vi "Release.vi"(8 "error in (no error)":errorcluster, 11 "SequenceCountService in":refnum<class "SequenceCountService.lvclass">) -> (0 "error out":errorcluster)   [LabVIEW 2020, in "Vecto.lvlib" / "SequenceCountService.lvclass"]
uses:
  SequenceCountService.lvclass
  SequenceCountService.lvclass/SequenceCountService.ctl
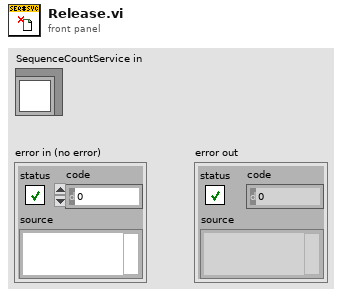
[diagram p1: front panel]
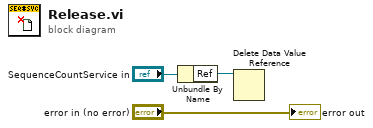
[diagram p0: block diagram]
diagram:
  n1 = Unbundle By Name("SequenceCountService in") -> ("Ref"=w2:refnum<data-value>)
  n2 = Delete Data Value Reference(data value reference=w2) -> ()  [unwired: 1 in, 2 out]
  "error out" <- "error in (no error)"
